vi "Create Statement Line with double quotes.vi"(8 "Error In":errorcluster) -> (0 "Error Out":errorcluster)   [LabVIEW 2018, in "Tests.lvlib"]
uses:
  Tests.lvlib
  src/Toolkit/Type Definitions/Statement.ctl
  src/Toolkit/Type Definitions/Tag.ctl
  src/Toolkit/Support/Create Level String.vi
  src/Toolkit/Support/Strip Whitespace.vi
  <vilib>/dlg_ctls.llb/Space Constant.vi
  <vilib>/Utility/error.llb/Trim Whitespace.vi
  <vilib>/addons/_JKI Toolkits/Caraya/classes/Test/Test.lvclass
  src/Toolkit/Toolkit.lvlib
  <vilib>/addons/_JKI Toolkits/Caraya/classes/Assert/Assert.lvclass
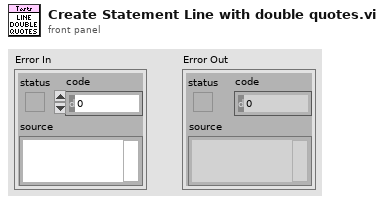
[diagram p1: front panel]
types:
  T1 = typedef "Toolkit.lvlib/Statement.ctl" = cluster{"Time Stamp":timestamp, "Tag":T2, "Source":string, "Message":string}
  T2 = typedef "Toolkit.lvlib/Tag.ctl" = enum16{"Fatal", "Error", "Warn", "Info", "Debug", "Trace"}
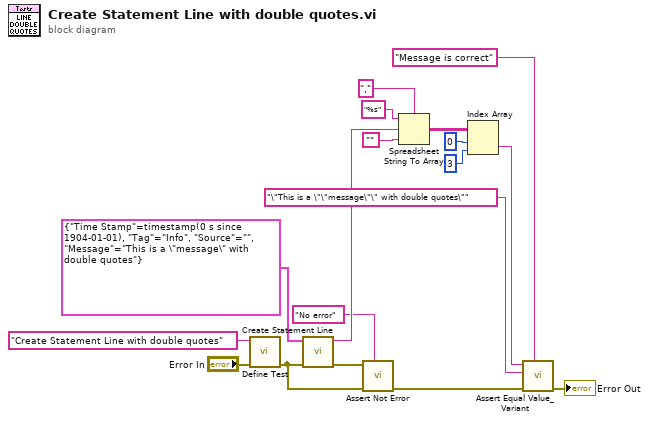
[diagram p0: block diagram]
diagram:
  n1 = call <vilib>:"Define Test.vi"("error in (no error)"="Error In", "Label (VI Title)"="Create Statement Line with double quotes") -> ("error out"=w7:errorcluster)  [unwired: 9 in]
  n2 = call "Create Statement Line.vi"("Error In"=w7, "Statement"=T1 {"Time Stamp"=timestamp(0 s since 1904-01-01), "Tag"=enum."Info", "Source"="", "Message"="This is a \"message\" with double quotes"}) -> ("Error Out"=w8:errorcluster, "Line"=w15:string)  [unwired: 8 in]
  n3 = call <vilib>:"Assert Not Error.vi"("Label"="No error", "error in (no error)"=w7, "Not Error?"=w8) -> ("error out"=w5:errorcluster)  [unwired: 8 in]
  n4 = Spreadsheet String To Array(delimiter (Tab)=",", format string="%s", spreadsheet string=w15, array type (2D Dbl)="") -> (array=w11:string[][])
  n5 = Index Array(array=w11, index (row)=0 ("disabled index (row)"), index (col)=3) -> (element=w1:string)
  n6 = call <vilib>:"Assert Equal Value_Variant.vi"("Label"="Message is correct", "error in (no error)"=w5, "Y"="\"This is a \"\"message\"\" with double quotes\"" ("Message"), "X"=w1) -> ("error out"=→"Error Out":errorcluster)  [unwired: 7 in]
